vi "Solve1.vi"(8 "Error In":errorcluster, 11 "object in":refnum<class "2021_2.lvclass">) -> (0 "Error Out":errorcluster, 2 "Result":u64, 3 "object out":refnum<class "2021_2.lvclass">)   [LabVIEW 2020, in "2021_2.lvclass"]
uses:
  2021_2.lvclass
  2021_2.lvclass/2021_2.ctl
panel:
  out "Depth":i32
  out "Forward":i32
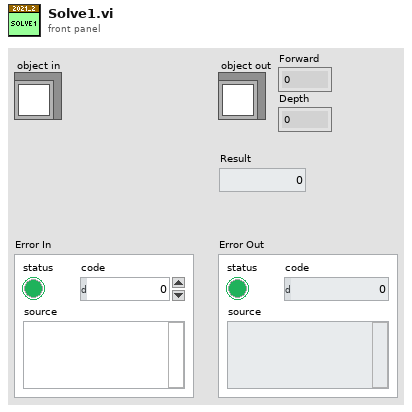
[diagram p1: front panel]
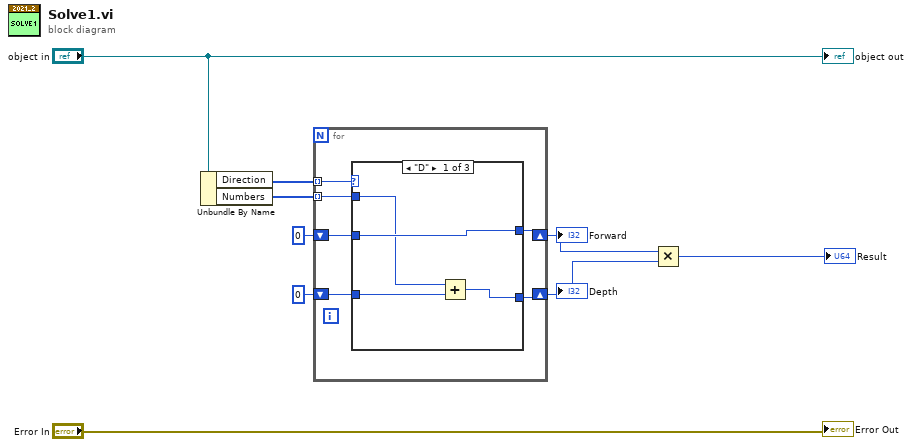
[diagram p0: block diagram]
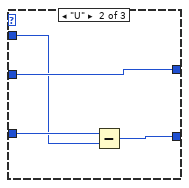
[diagram p2: hidden frame]
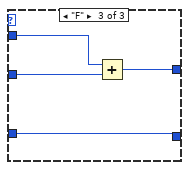
[diagram p3: hidden frame]
diagram:
  n1 = Unbundle By Name("object in") -> ("Direction"=w4:enum16{"F", "D", "U"}[], "Numbers"=w6:i32[])
  n2 = for {
    tunnel: w6 -> [w10] mode=indexing
    shift-right: [w14] -> w1
    shift-left: 0 -> [w15]
    tunnel: w4 -> [w13] mode=indexing
    shift-right: [w12] -> w2
    shift-left: 0 -> [w11]
    n3 = case shown="\"D\"" w13 {
      tunnel: w15 -> [w19 w23 w25]
      tunnel: [w18 w22 w25] -> w14
      tunnel: w11 -> [w17 w21 w26]
      tunnel: [w17 w21 w27] -> w12
      tunnel: w10 -> [w16 w20 w24]
      frame "D" {
        n4 = Add(x=w16, y=w19) -> (x+y=w18:i32)
      }
      frame "U" {
        n5 = Subtract(x=w23, y=w20) -> (x-y=w22:i32)
      }
      frame "F" {
        n6 = Add(x=w24, y=w26) -> (x+y=w27:i32)
      }
    }
  }
  "Forward" <- w2
  "Depth" <- w1
  n7 = Multiply(x=w2, y=w1) -> (x*y=→"Result":i32)
  "Error Out" <- "Error In"
  "object out" <- "object in"
